vi "Update Time Remaining.vi"(8 "error in (no error)":errorcluster, 10 "Timing":dbl, 11 "Simulated Wash Display Console Actor in":refnum<class "Simulated Wash Display Console Actor.lvclass">) -> (0 "error out":errorcluster, 3 "Simulated Wash Display Console Actor out":refnum<class "Simulated Wash Display Console Actor.lvclass">)   [LabVIEW 2019, in "Simulated Wash Display Console Actor.lvlib" / "Simulated Wash Display Console Actor.lvclass"]
uses:
  Simulated Wash Display Console Actor.lvclass
  Simulated Wash Display Console Actor.lvclass/Simulated Wash Display Console Actor.ctl
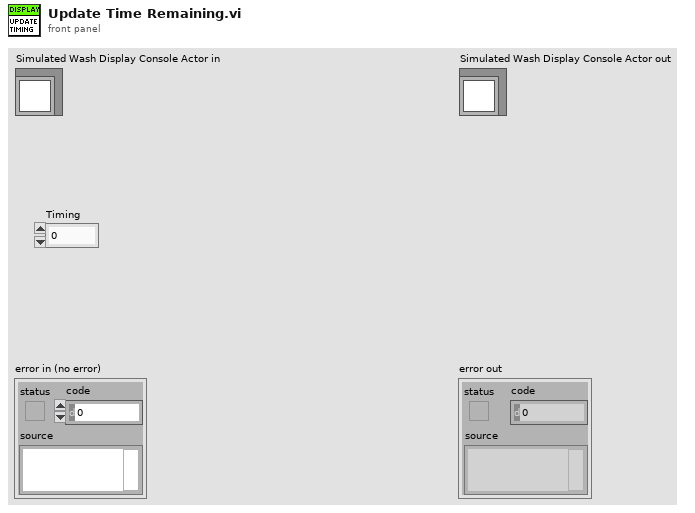
[diagram p1: front panel]
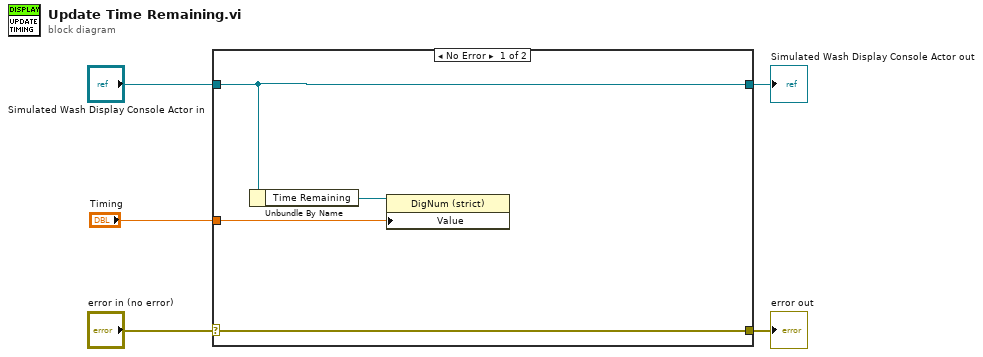
[diagram p0: block diagram]
diagram:
  n1 = case shown="No Error" "error in (no error)" {
    selector: "error in (no error)" -> [w9 w10]
    tunnel: [w9 w10] -> w4
    tunnel: [w6 w11] -> w2
    tunnel: "Simulated Wash Display Console Actor in" -> [w6 w11]
    tunnel: "Timing" -> [w7 _]
    frame No Error {
      n2 = Unbundle By Name(w6) -> ("Time Remaining"=w8:refnum<vi>)
      n3 = property class="DigNum (strict)"(reference=w8, "Value"=w7) -> ()  [unwired: 1 in, 2 out]
    }
    frame Error {
    }
  }
  "error out" <- w4
  "Simulated Wash Display Console Actor out" <- w2
